vi "Bound and Position to Rect-Bound.vi"(3 "Position":T2, 5 "Bounds":T1) -> (1 "Rect Bound":T3)   [LabVIEW 2017]
doc: "Converts a Position (Left, Top) and a Bounds (Width, Height) into a LabVIEW Rect cluster holding the left, top, right and bottom edges."
uses:
  <vilib>/Utility/miscctls.llb/LVPositionTypeDef.ctl
  <vilib>/Utility/miscctls.llb/LVBoundsTypeDef.ctl
  <vilib>/Utility/miscctls.llb/LVRectTypeDef.ctl
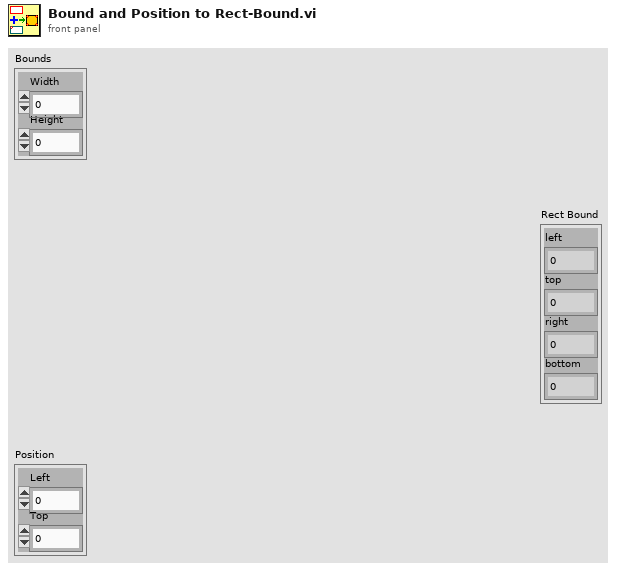
[diagram p1: front panel]
types:
  T1 = typedef "LVBoundsTypeDef.ctl" = cluster{"Width":u32, "Height":u32}
  T2 = typedef "LVPositionTypeDef.ctl" = cluster{"Left":i32, "Top":i32}
  T3 = cluster{"left":i16, "top":i16, "right":i16, "bottom":i16}
  T4 = typedef "LVRectTypeDef.ctl" = cluster{"Left":i16, "Top":i16, "Right":i16, "Bottom":i16}
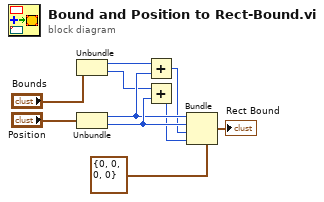
[diagram p0: block diagram]
diagram:
  n1 = Unbundle("Bounds") -> ("Width"=w4:u32, "Height"=w5:u32)
  n2 = Unbundle("Position") -> ("Left"=w8:i32, "Top"=w9:i32)
  n3 = Add(x=w4, y=w8) -> (x+y=w6:u32)
  n4 = Add(x=w5, y=w9) -> (x+y=w7:u32)
  n5 = Bundle(cluster=T4 {"Left"=0, "Top"=0, "Right"=0, "Bottom"=0} ("Windows Bounds"), "Left"=w8, "Top"=w9, "Right"=w6, "Bottom"=w7) -> (→"Rect Bound":T4)
